vi "LVDimInterface.dim_unfold_data.vi"(0 "rawData":i8[](array[numeric]), 5 "error in (no error)":errorcluster) -> (14 "data":i8[](array[numeric]), 15 "callBackID":i32, 17 "no link":bool, 19 "error out":errorcluster)   [LabVIEW 2014, in "LVDimInterface.lvlib"]
doc: "Unfolds the data from the DIMWrapper dll.\n\nHistory: 13-FEB-2006, Dietrich Beck\n\nCopyright (C)\nGesellschaft für Schwerionenforschung, GSI\nPlanckstr. 1\n64291 Darmstadt\nGermany\n\nContact: D.Beck@gsi.de \n\nThis program is free software; you can redistribute it and/or modify it under the terms of the \nGNU General Public License as published by the Free Software Foundation; either version 2 of the license, or (at your option) any later version.\n\nThis program is distributed in the hope that it will be useful, but WITHOUT ANY WARRANTY; without even the implied warranty of MERCHANTABILITY or FITNESS FOR A PARTICULAR PURPOSE. See the GNU General License for more details (http://www.gnu.org).\n\nGesellschaft für Schwerionenforschung, GSI\nPlanckstr. 1, 64291 Darmstadt, Germany\nFor all questions and ideas contact D. Beck.\nLast update: 16-DEC-2005"
uses:
  LVDimInterface.lvlib
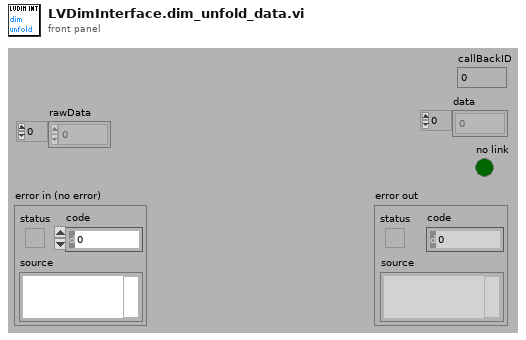
[diagram p1: front panel]
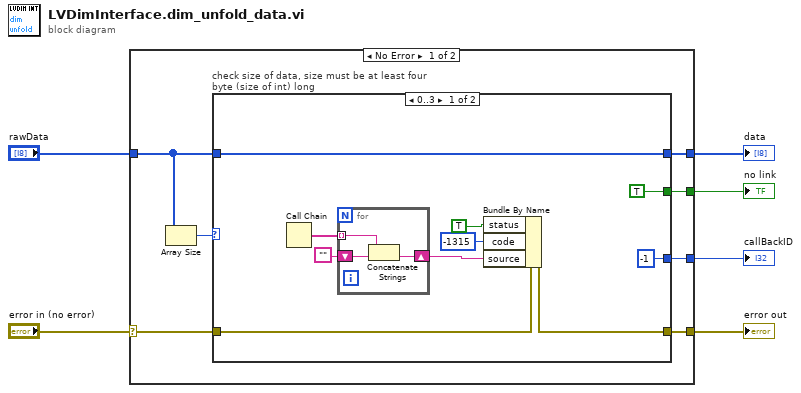
[diagram p0: block diagram]
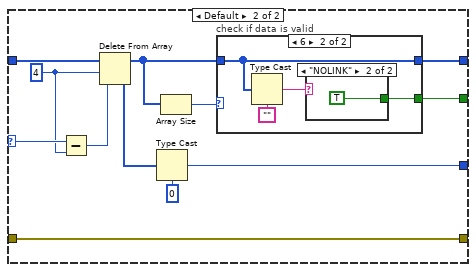
[diagram p2: hidden frame]
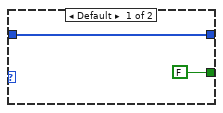
[diagram p3: hidden frame]
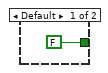
[diagram p4: hidden frame]
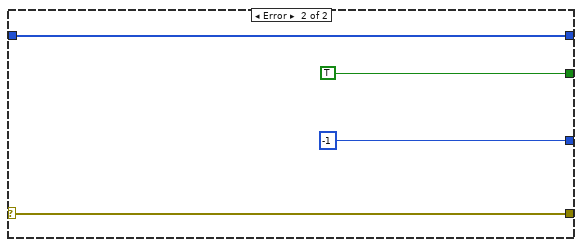
[diagram p5: hidden frame]
diagram:
  n1 = case shown="No Error" "error in (no error)" {
    selector: "error in (no error)" -> [w12 w50]
    tunnel: [w13 w50] -> w6
    tunnel: "rawData" -> [w10 w49]
    tunnel: [w9 w49] -> w3
    tunnel: [w8 -1 ("callBackID (out)")] -> w2
    tunnel: [w7 TRUE] -> w1
    frame No Error {
      n2 = Array Size(array=w10) -> (size(s)=w11:i32)
      n3 = case "check size of data, size must be at least four byte (size of int) long" shown="0..3" w11 {
        selector: w11 -> [_ w37]
        tunnel: w12 -> [w19 w31]
        tunnel: [w18 w31] -> w13
        tunnel: w10 -> [w16 w38]
        tunnel: [w16 w28] -> w9
        tunnel: [-1 w32] -> w8
        tunnel: [TRUE w27] -> w7
        frame 0..3 {
          n4 = Call Chain() -> (call chain=w22:string[])
          n5 = for {
            tunnel: w22 -> [w24] mode=indexing
            shift-right: [w26] -> w20
            shift-left: "" ("Empty String Constant") -> [w25]
            n6 = Concatenate Strings(w24, w25) -> (w26:string)
          }
          n7 = Bundle By Name(cluster=w19, "status"=TRUE, "code"=-1315, "source"=w20) -> (w18:errorcluster)
        }
        frame Default {
          w36 = 4 ("length")
          n8 = Subtract(x=w37, y=w36) -> (x-y=w35:i32)
          n9 = Delete From Array(array=w38, length=w36, index=w35) -> (deleted portion=w34:i8[], array with subset deleted=w29:i8[])
          n10 = Type Cast(type=0, x=w34) -> (*(type *) &x=w32:i32)
          n11 = Array Size(array=w29) -> (size(s)=w30:i32)
          n12 = case "check if data is valid" shown="6" w30 {
            tunnel: [w40 w42] -> w28
            tunnel: w29 -> [w40 w42]
            tunnel: [FALSE w41] -> w27
            frame Default {
            }
            frame 6 {
              n13 = Type Cast(type="" ("Empty String Constant"), x=w42) -> (*(type *) &x=w43:string)
              n14 = case shown="\"NOLINK\"" w43 {
                tunnel: [FALSE TRUE] -> w41
                frame Default {
                }
                frame "NOLINK" {
                }
              }
            }
          }
        }
      }
    }
    frame Error {
    }
  }
  "error out" <- w6
  "data" <- w3
  "callBackID" <- w2
  "no link" <- w1
